vi "main003.vi"() -> ()   [LabVIEW 2015]
uses:
  <vilib>/DAQmx/write.llb/DAQmx Write (Analog DBL 1Chan 1Samp).vi
  <vilib>/DAQmx/miscellaneous.llb/DAQmx Fill In Error Info.vi
  <vilib>/DAQmx/create/channels.llb/DAQmx Create Channel (AO-Voltage-Basic).vi
  subvi/Newport ESP301/Newport ESP301.lvlib
panel:
  out "speed":dbl(graph)
  in  "pump_waypoints":string[][](table)
  in  "Boolean":bool
  out "a":waveform(dbl)(graph)={"t0"=timestamp(3620209335.8073797 s since 1904-01-01), "dt"=1.0, "Y"=[nan]}
  out "Waveform Chart":dbl(graph)=5.25341140860948
  in  "physical channels":tag="Dev3/ao1"
  out "DAC error":errorcluster
  out "ESP error":errorcluster={"status"=TRUE, "code"=-1073807343, "source"="VISA Open in Newport ESP301.lvlib:Initialize.vi->main002.vi"}
  out "run?":bool
  in  "set_vel":bool
  in  "velocity [fs/s]":dbl=667.128190396304
  in  "vel_mm":dbl caption="velocity [mm/s]"
  out "meas. velocity":dbl=nan
  in  "stop":bool
  out "output voltage":dbl=nan
  in  "start":bool
  in  "go2p1":bool
  out "position [fs]":dbl=nan
  out "position [mm]":dbl=nan
  in  "p2 [mm]":dbl=2.0
  in  "p1 [mm]":dbl
  in  "interpolate output":bool
  in  "t2 [fs]":dbl=6671.281903963041
  in  "t1 [fs]":dbl=-6671.281903963041
  in  "t0 [mm]":dbl=1.0
  in  "Axis (1)":i32=2 min=1 max=3
  in  "Serial Link (RS232)":enum16{"RS232", "USB"}(ring)
  in  "VISA resource name":refnum<visa-resource-name>="COM9"
  in  "main_close":bool
  # "Always use CLOSE button to correctly disconnect the device. STOP program afterwards."
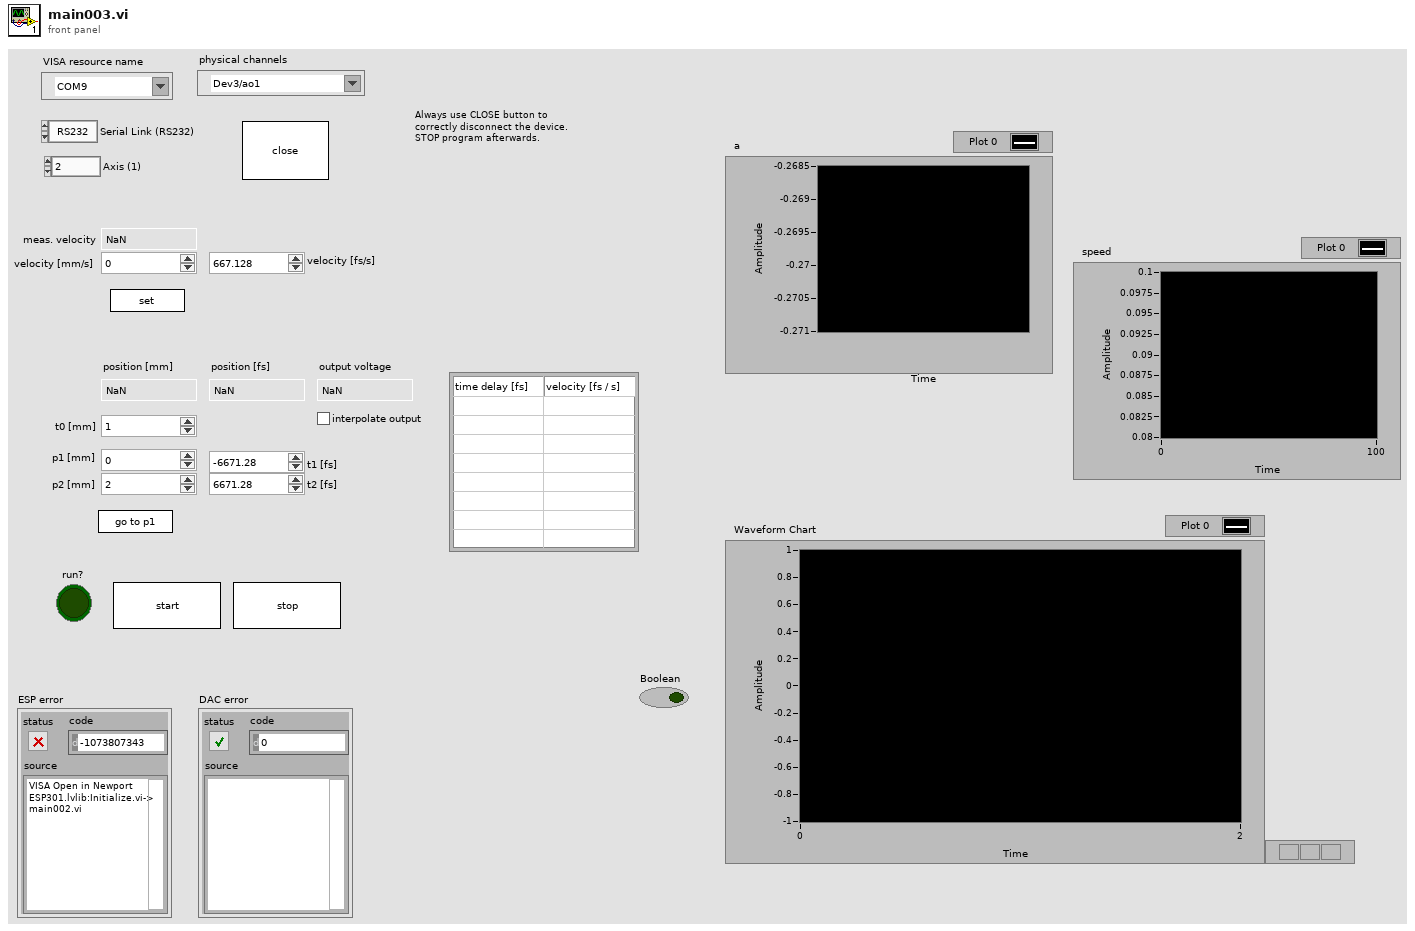
[diagram p1: front panel]
types:
  T1 = cluster{"dev1_data":refnum<queue>, "dev2_data":refnum<queue>}
  T2 = cluster{"dev1_cmd":refnum<queue>, "dev2_cmd":refnum<queue>}
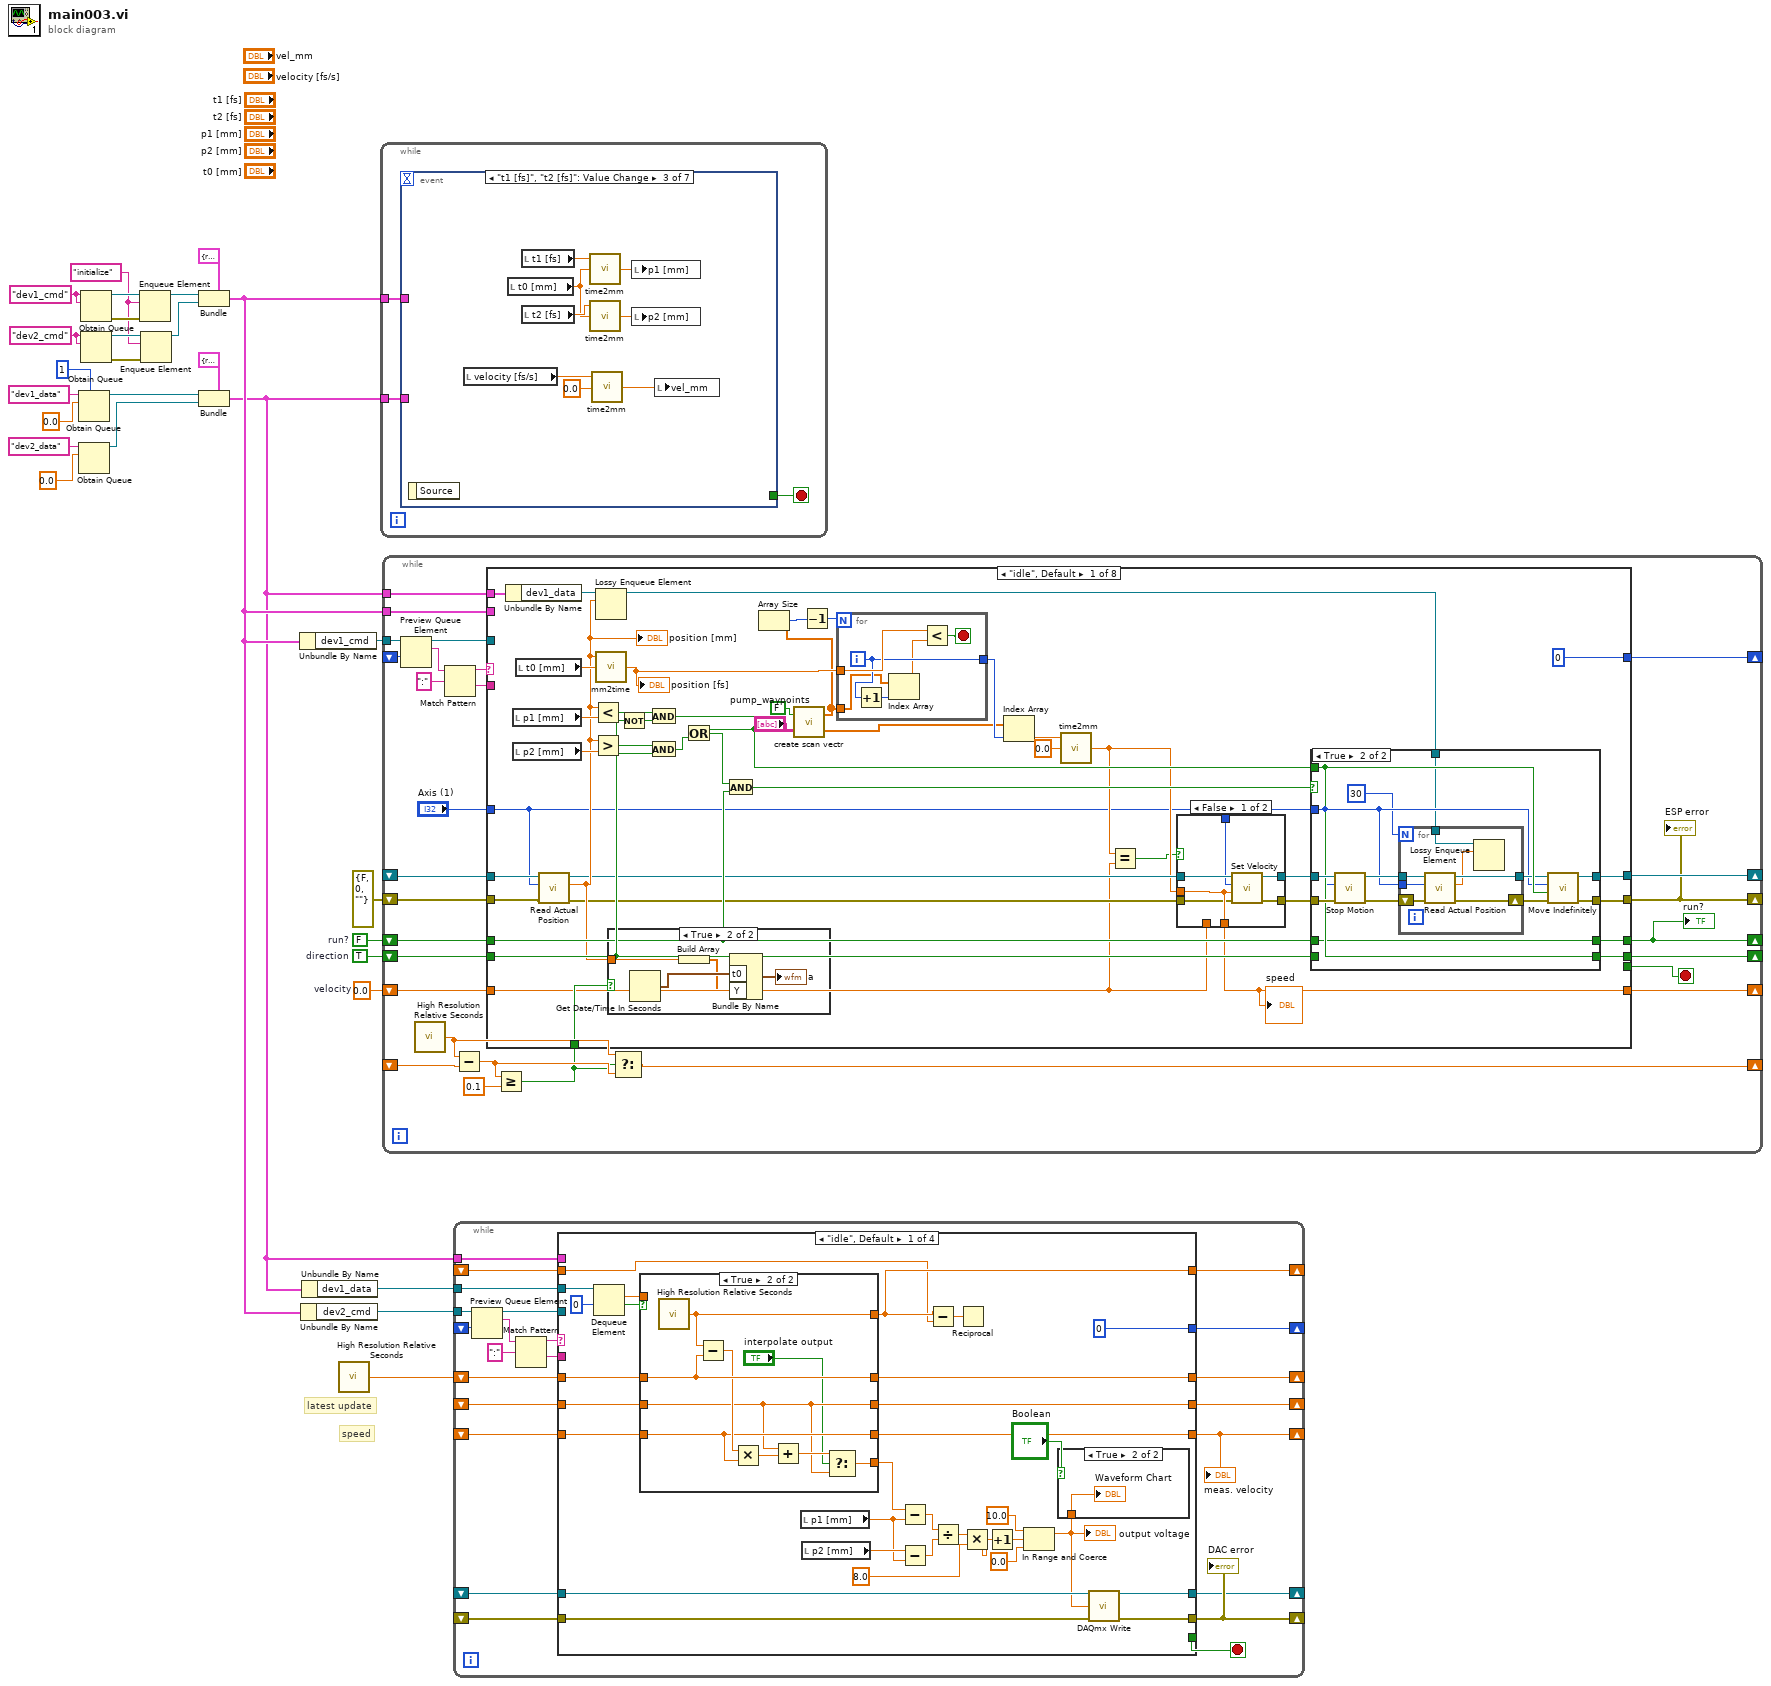
[diagram p0: block diagram]
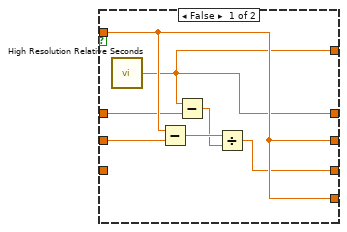
[diagram p3: hidden frame]
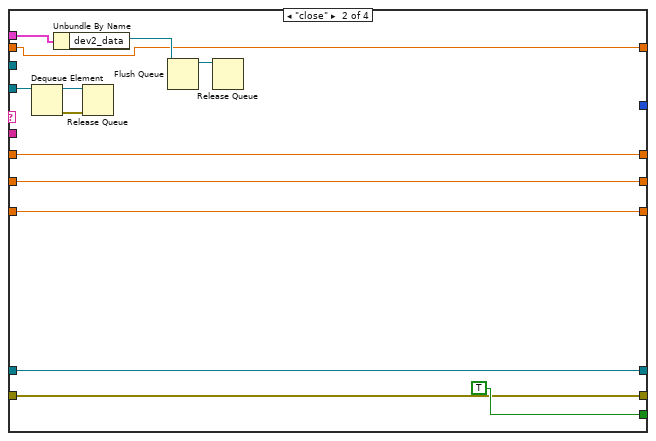
[diagram p4: hidden frame]
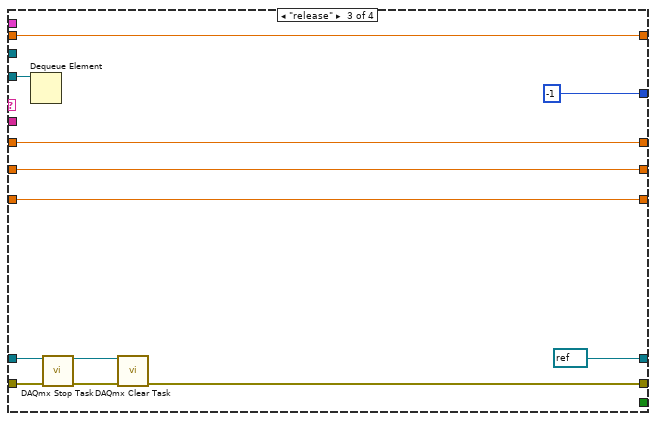
[diagram p5: hidden frame]
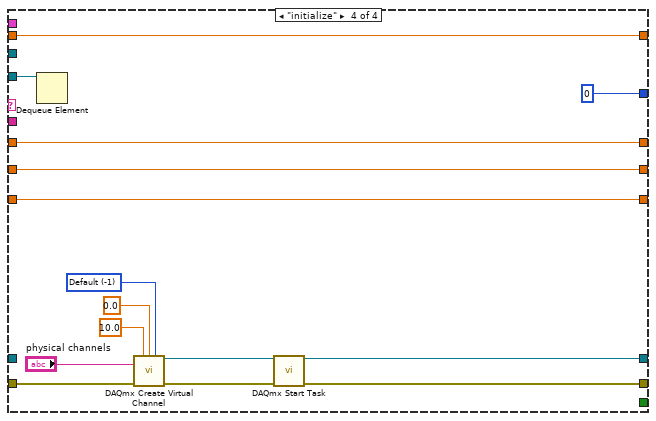
[diagram p6: hidden frame]
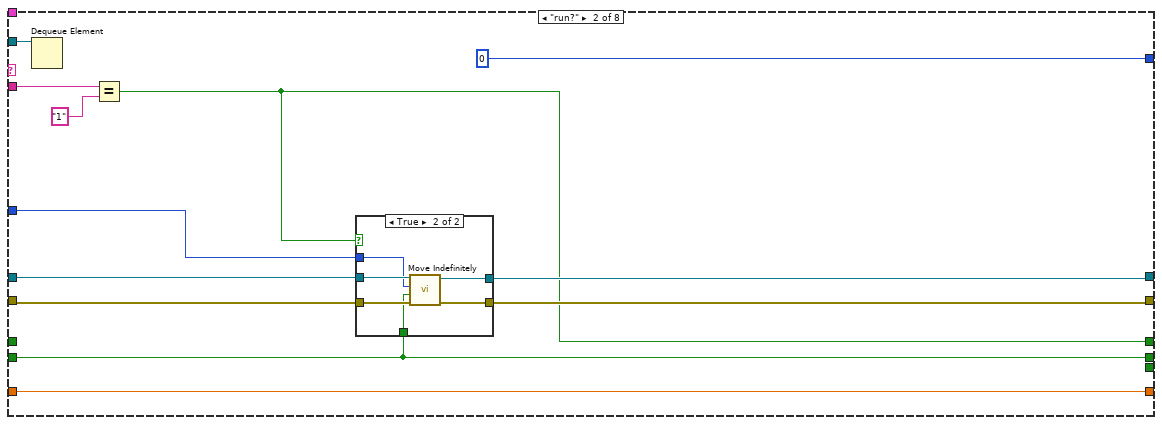
[diagram p10: hidden frame]
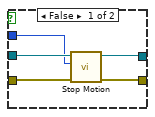
[diagram p11: hidden frame]
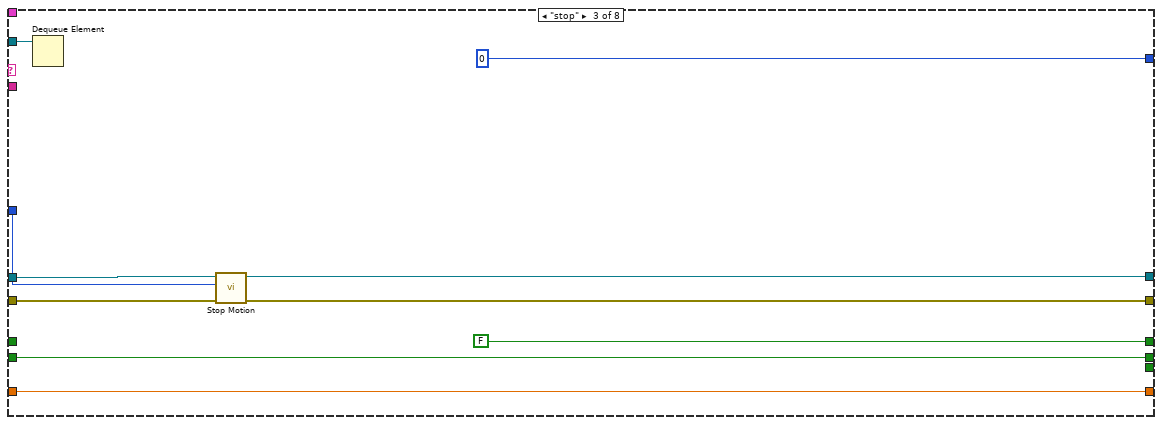
[diagram p12: hidden frame]
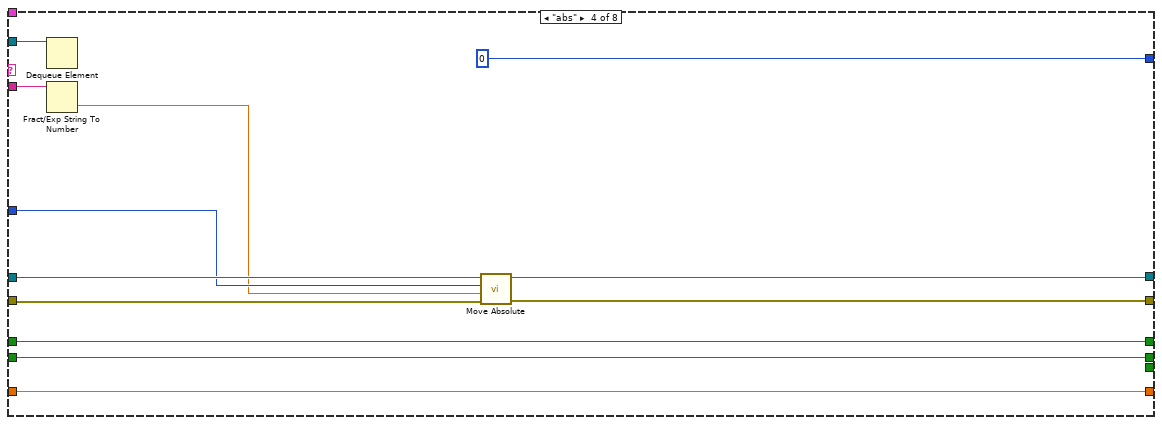
[diagram p13: hidden frame]
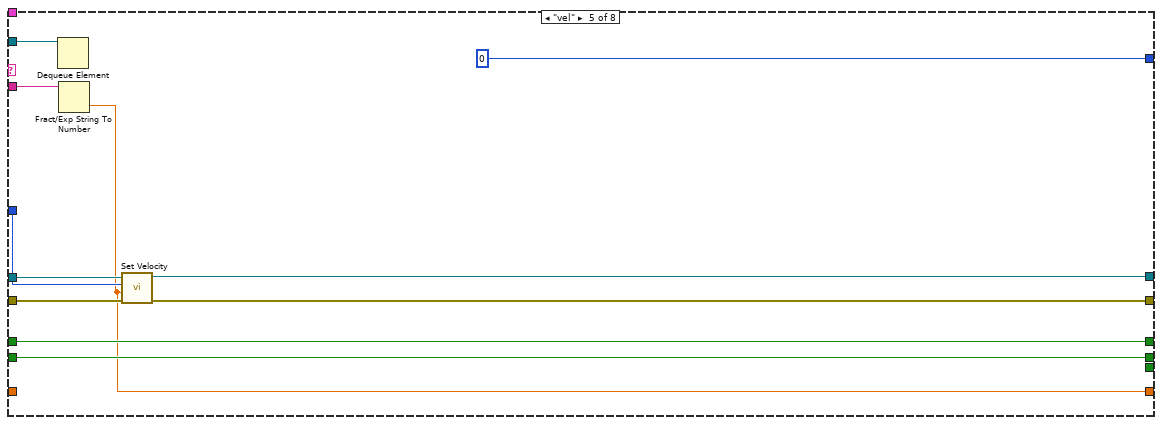
[diagram p14: hidden frame]
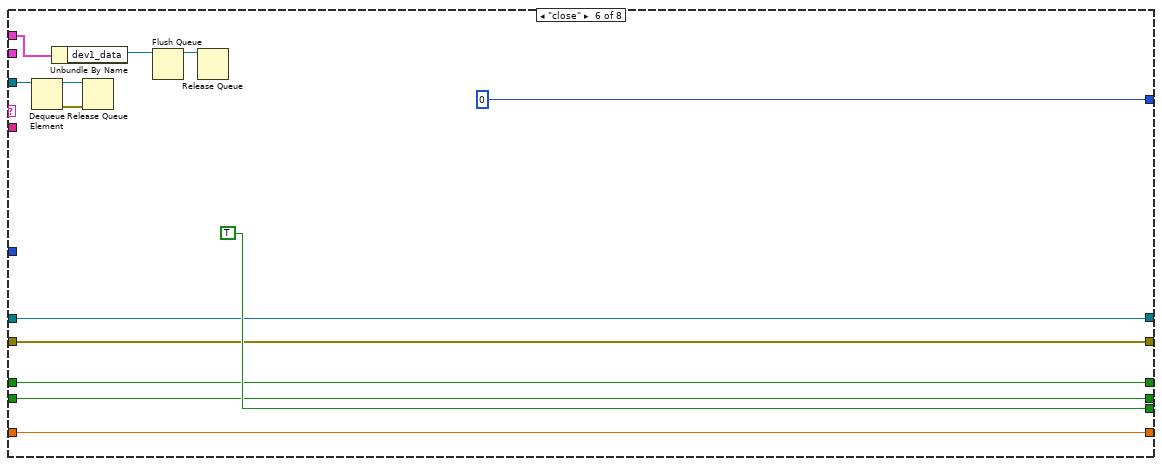
[diagram p15: hidden frame]
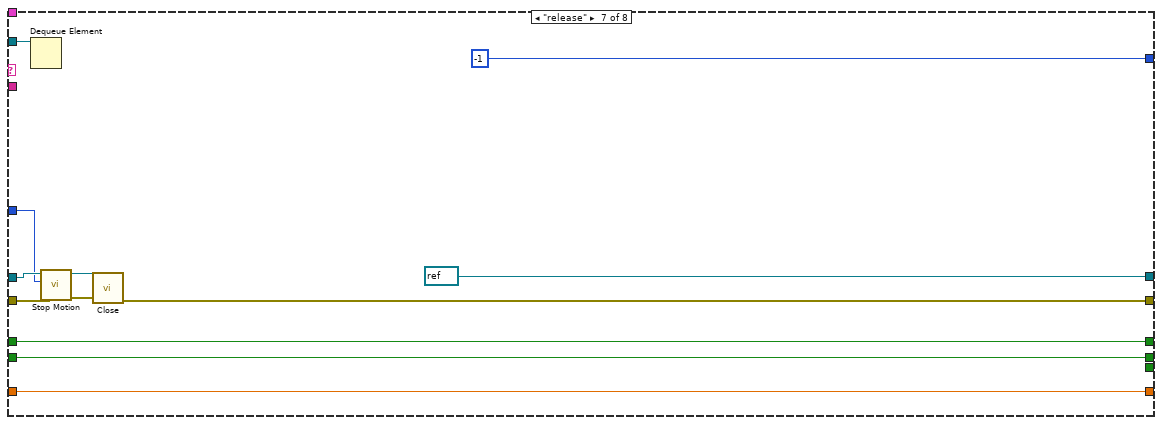
[diagram p16: hidden frame]
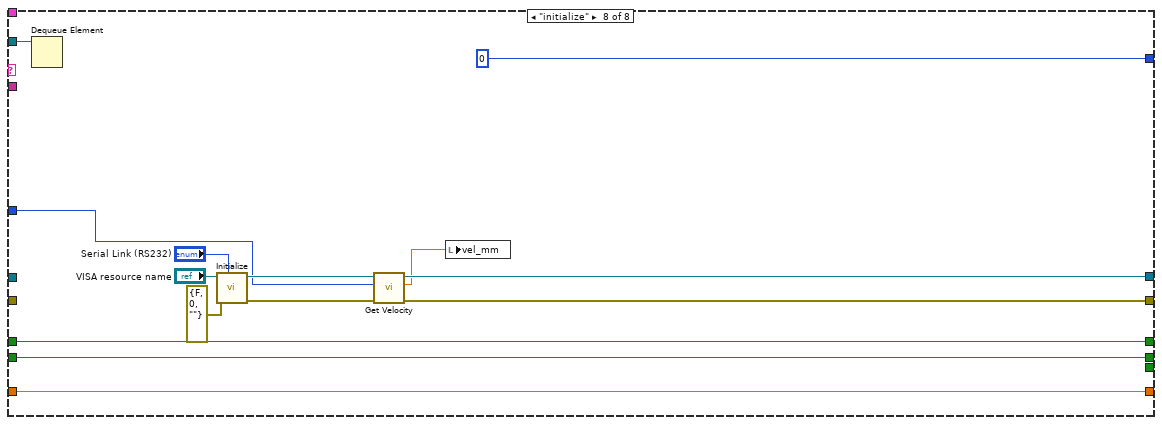
[diagram p17: hidden frame]
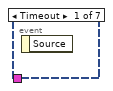
[diagram p18: hidden frame]
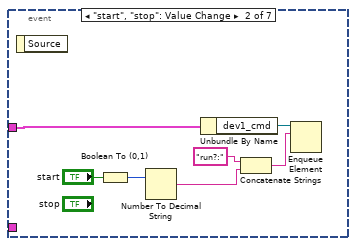
[diagram p19: hidden frame]
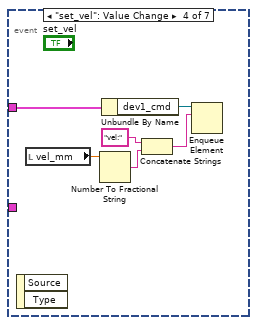
[diagram p20: hidden frame]
diagram:
  w1 = 0.0  # velocity
  w2 = TRUE  # direction
  w5 = FALSE  # run?
  w16 = "dev2_cmd" ("name (unnamed)")
  w22 = "initialize" ("element")
  w17 = "dev1_cmd" ("name (unnamed)")
  # "speed"
  # "latest update"
  n1 = Obtain Queue(max queue size (-1, unlimited)=1, name (unnamed)="dev1_data", element data type=0.0) -> (queue out=w13:refnum<queue>)  [unwired: 2 in, 2 out]
  n2 = Obtain Queue(name (unnamed)="dev2_data", element data type=0.0) -> (queue out=w12:refnum<queue>)  [unwired: 3 in, 2 out]
  n3 = Obtain Queue(name (unnamed)=w17, element data type=w17) -> (queue out=w28:refnum<queue>, error out=w27:errorcluster)  [unwired: 3 in, 1 out]
  n4 = Obtain Queue(name (unnamed)=w16, element data type=w16) -> (queue out=w23:refnum<queue>, error out=w24:errorcluster)  [unwired: 3 in, 1 out]
  n5 = Enqueue Element(queue=w28, element=w22, error in (no error)=w27) -> (queue out=w25:refnum<queue>)  [unwired: 1 in, 2 out]
  n6 = Enqueue Element(queue=w23, element=w22, error in (no error)=w24) -> (queue out=w21:refnum<queue>)  [unwired: 1 in, 2 out]
  n7 = Bundle(cluster=T2 {"dev1_cmd"=refnum, "dev2_cmd"=refnum}, "dev1_cmd"=w25, "dev2_cmd"=w21) -> (w9:T2)
  n8 = Bundle(cluster=T1 {"dev1_data"=refnum, "dev2_data"=refnum}, "dev1_data"=w13, "dev2_data"=w12) -> (w3:T1)
  n9 = Unbundle By Name(w9) -> ("dev1_cmd"=w18:refnum<queue>)
  n10 = Unbundle By Name(w9) -> ("dev2_cmd"=w8:refnum<queue>)
  n11 = Unbundle By Name(w3) -> ("dev1_data"=w7:refnum<queue>)
  n12 = call <vilib>:"High Resolution Relative Seconds.vi"() -> ("relative seconds"=w6:dbl)
  n13 = while {
    tunnel: w9 -> [w31]
    tunnel: w3 -> [w30]
    stop <- w29 stop-if-true
    n14 = event shown="[2] \"t1 [fs]\", \"t2 [fs]\": Value Change" {
      selector: _ -> [_ _ _ _ _ _ _]
      dyn-events: _ -> [_ _ _ _ _ _ _]
      timeout: _ -> [_ _ _ _ _ _ _]
      tunnel: w31 -> [_ w35 _ w48 _ w66 w69]
      tunnel: w30 -> [_ _ _ _ _ _ _]
      tunnel: [_ _ _ _ _ _ TRUE] -> w29
      event Timeout {
        n15 = event-data() -> ()  [unwired: 1 in, 1 out]
      }
      event "start", "stop": Value Change {
        n16 = event-data() -> ()  [unwired: 1 in, 1 out]
        n17 = Boolean To (0,1)(Boolean="start") -> (0, 1=w33:i16)
        n18 = Number To Decimal String(number=w33) -> (decimal integer string=w32:string)  [unwired: 1 in]
        n19 = Unbundle By Name(w35) -> ("dev1_cmd"=w38:refnum<queue>)
        n20 = Concatenate Strings("run?:" ("string"), w32) -> (w37:string)
        n21 = Enqueue Element(queue=w38, element=w37) -> ()  [unwired: 2 in, 3 out]
      }
      event "t1 [fs]", "t2 [fs]": Value Change {
        n22 = event-data() -> ()  [unwired: 1 in, 1 out]
        n23 = local read "velocity [fs/s]"() -> (w41:dbl)
        n24 = local read "t0 [mm]"() -> (w44:dbl)
        n25 = local read "t1 [fs]"() -> (w45:dbl)
        n26 = local read "t2 [fs]"() -> (w46:dbl)
        n27 = call "time2mm.vi"("Offset (mm)"=w44, "time"=w45) -> ("position (mm)"=w42:dbl)  [unwired: 1 in]
        n28 = call "time2mm.vi"("Offset (mm)"=w44, "time"=w46) -> ("position (mm)"=w43:dbl)  [unwired: 1 in]
        n29 = call "time2mm.vi"("Offset (mm)"=0.0, "time"=w41) -> ("position (mm)"=w39:dbl)  [unwired: 1 in]
        n30 = local write "p1 [mm]"(w42) -> ()
        n31 = local write "p2 [mm]"(w43) -> ()
        n32 = local write "vel_mm"(w39) -> ()
      }
      event "set_vel": Value Change {
        n33 = event-data() -> ()  [unwired: 1 in, 2 out]
        n34 = local read "vel_mm"() -> (w47:dbl)
        n35 = Number To Fractional String(number=w47) -> (F-format string=w51:string)  [unwired: 3 in]
        n36 = Unbundle By Name(w48) -> ("dev1_cmd"=w52:refnum<queue>)
        n37 = Concatenate Strings("vel:" ("string"), w51) -> (w50:string)
        n38 = Enqueue Element(queue=w52, element=w50) -> ()  [unwired: 2 in, 3 out]
      }
      event "p1 [mm]", "p2 [mm]", "t0 [mm]", "vel_mm": Value Change {
        n39 = event-data() -> ()  [unwired: 1 in, 2 out]
        n40 = local read "vel_mm"() -> (w55:dbl)
        n41 = local read "p1 [mm]"() -> (w59:dbl)
        n42 = local read "p2 [mm]"() -> (w60:dbl)
        n43 = local read "t0 [mm]"() -> (w58:dbl)
        n44 = call "mm2time.vi"("Offset (mm)"=w58, "distance (mm)"=w59) -> ("time in fs"=w56:dbl)  [unwired: 1 in]
        n45 = call "mm2time.vi"("Offset (mm)"=w58, "distance (mm)"=w60) -> ("time in fs"=w57:dbl)  [unwired: 1 in]
        n46 = call "mm2time.vi"("Offset (mm)"=0.0, "distance (mm)"=w55) -> ("time in fs"=w54:dbl)  [unwired: 1 in]
        n47 = local write "t1 [fs]"(w56) -> ()
        n48 = local write "t2 [fs]"(w57) -> ()
        n49 = local write "velocity [fs/s]"(w54) -> ()
      }
      event "go2p1": Value Change {
        n50 = event-data() -> ()  [unwired: 1 in, 2 out]
        n51 = local read "p1 [mm]"() -> (w61:dbl)
        n52 = Number To Fractional String(number=w61) -> (F-format string=w64:string)  [unwired: 3 in]
        n53 = Unbundle By Name(w66) -> ("dev1_cmd"=w65:refnum<queue>)
        n54 = Concatenate Strings("abs:" ("string"), w64) -> (w62:string)
        n55 = Enqueue Element(queue=w65, element=w62) -> ()  [unwired: 2 in, 3 out]
      }
      event "main_close": Value Change {
        n56 = event-data() -> ()  [unwired: 1 in, 1 out]
        n57 = Cluster To Array(cluster=w69) -> (array=w68:refnum<queue>[])
        n58 = for {
          tunnel: w68 -> [w74] mode=indexing
          n59 = Flush Queue(queue=w74) -> (queue out=w70:refnum<queue>)  [unwired: 1 in, 2 out]
          n60 = Enqueue Element(queue=w70, element="release") -> (queue out=w72:refnum<queue>)  [unwired: 2 in, 2 out]
          n61 = Enqueue Element(queue=w72, element="close") -> ()  [unwired: 2 in, 3 out]
        }
      }
    }
  }
  n62 = while {
    tunnel: w9 -> [w97]
    tunnel: w18 -> [w102]
    tunnel: w3 -> [w94]
    shift-right: [w92] -> _
    shift-left: _ -> [w93]
    shift-right: [w91] -> _
    shift-left: _ -> [w88]
    shift-right: [w90] -> _
    shift-left: errorcluster {"status"=FALSE, "code"=0, "source"=""} ("error out") -> [w89]
    shift-right: [w85] -> _
    shift-left: w5 -> [w86]
    shift-right: [w83] -> _
    shift-left: w2 -> [w84]
    shift-right: [w77] -> _
    shift-left: _ -> [w82]
    shift-right: [w75] -> _
    shift-left: w1 -> [w76]
    stop <- w95 stop-if-true
    n63 = Preview Queue Element(queue=w102, timeout in ms (-1)=w93) -> (queue out=w96:refnum<queue>, element=w101:string)  [unwired: 1 in, 2 out]
    n64 = call <vilib>:"High Resolution Relative Seconds.vi"() -> ("relative seconds"=w79:dbl)
    n65 = Match Pattern(string=w101, regular expression=":") -> (before substring=w99:string, after substring=w98:string)  [unwired: 1 in, 2 out]
    n66 = Subtract(x=w79, y=w82) -> (x-y=w80:dbl)
    n67 = Greater Or Equal?(x=w80, y=0.1) -> (x >= y?=w78:bool)
    n68 = case shown="\"idle\", Default" w99 {
      tunnel: w98 -> [_ w200 _ w232 w239 _ _ _]
      tunnel: w97 -> [_ _ _ _ _ _ _ _]
      tunnel: w96 -> [_ w198 w214 w233 w238 w257 w268 w279]
      tunnel: [_ _ _ _ _ TRUE _ _] -> w95
      tunnel: w94 -> [w144 _ _ _ _ w249 _ _]
      tunnel: [0 0 0 0 0 0 -1 0] -> w92
      tunnel: [w119 w195 w219 w229 w244 w253 refnum<visa-resource-name> refnum ("VISA resource name out") w275] -> w91
      tunnel: [w114 w194 w218 w228 w243 w252 w267 w274] -> w90
      tunnel: w89 -> [w140 w192 w220 w230 w242 w252 w263 _]
      tunnel: w88 -> [w141 w193 w221 w231 w241 w253 w260 _]
      tunnel: "Axis (1)" -> [w108 w196 w217 w227 w240 _ w259 w276]
      tunnel: w86 -> [w129 _ _ w224 w236 w250 w265 w280]
      tunnel: [w128 w191 FALSE ("run?") w224 w236 w250 w265 w280] -> w85
      tunnel: w84 -> [w130 w190 w213 w223 w235 w246 w264 w271]
      tunnel: [w131 w190 w213 w223 w235 w246 w264 w271] -> w83
      tunnel: w78 -> [w127 _ _ _ _ _ _ _]
      tunnel: w76 -> [w113 w189 w212 w222 _ w245 w258 w270]
      tunnel: [w106 w189 w212 w222 w234 w245 w258 w270] -> w75
      frame "idle", Default {
        n69 = Unbundle By Name(w144) -> ("dev1_data"=w143:refnum<queue>)
        n70 = local read "p1 [mm]"() -> (w139:dbl)
        n71 = local read "p2 [mm]"() -> (w138:dbl)
        n72 = local read "t0 [mm]"() -> (w142:dbl)
        n73 = call "Read Actual Position.vi"("error in (no error)"=w140, "Axis (1)"=w108, "VISA resource name"=w141) -> ("error out"=w115:errorcluster, "Position (units)"=w126:dbl, "VISA resource name out"=w118:refnum<visa-resource-name>)  [unwired: 2 in]
        "position [mm]" <- w126
        n74 = Less?(x=w126, y=w139) -> (x < y?=w136:bool)
        n75 = Greater?(x=w126, y=w138) -> (0:w135:bool)
        n76 = Lossy Enqueue Element(queue=w143, element=w126) -> (queue out=w125:refnum<queue>)  [unwired: 1 in, 3 out]
        n77 = call "mm2time.vi"("Offset (mm)"=w142, "distance (mm)"=w126) -> ("time in fs"=w120:dbl)  [unwired: 1 in]
        "position [fs]" <- w120
        n78 = case shown="True" w127 {
          tunnel: w126 -> [_ w164]
          frame False {
          }
          frame True {
            n79 = Get Date/Time In Seconds() -> (seconds since 1Jan1904=w163:timestamp)
            n80 = Build Array(w164) -> (w162:dbl[])
            n81 = Bundle By Name("t0"=w163, "Y"=w162) -> (→"a":waveform(dbl))  [unwired: 1 in]
          }
        }
        n82 = Not(x=w130) -> (.not. x?=w137:bool)
        n83 = And(x=w136, y=w137) -> (x .and. y?=w132:bool)
        n84 = And(x=w135, y=w130) -> (x .and. y?=w134:bool)
        n85 = Or(x=w132, y=w134) -> (x .or. y?=w133:bool)
        n86 = And(x=w133, y=w129) -> (x .and. y?=w112:bool)
        n87 = call "create scan vectr.vi"("Table Control"="pump_waypoints", "waypoint mode?"=FALSE) -> ("Array 2"=w123:dbl[], "Array"=w105:dbl[])
        n88 = Array Size(array=w105) -> (size(s)=w103:i32)
        n89 = Decrement(x=w103) -> (x-1=w104:i32)
        n90 = for {
          N: w104 -> [_]
          tunnel: w105 -> [w155]
          tunnel: w120 -> [w160]
          tunnel: [w157] -> w124
          i -> [w157]
          stop <- w159 stop-if-true
          n91 = Increment(x=w157) -> (x+1=w158:i32)
          n92 = Index Array(array=w155, index=w158) -> (element=w156:dbl)
          n93 = Less?(x=w160, y=w156) -> (x < y?=w159:bool)
        }
        n94 = Index Array(array=w123, index=w124) -> (element=w111:dbl)
        n95 = call "time2mm.vi"("Offset (mm)"=0.0, "time"=w111) -> ("position (mm)"=w109:dbl)  [unwired: 1 in]
        n96 = Equal?(x=w109, y=w113) -> (x = y?=w107:bool)
        n97 = case shown="False" w107 {
          tunnel: w118 -> [w148 w154]
          tunnel: [w151 w154] -> w117
          tunnel: [w150 w153] -> w116
          tunnel: w115 -> [w146 w153]
          tunnel: w113 -> [_ w152]
          tunnel: [w149 w152] -> w106
          tunnel: w109 -> [w149 _]
          tunnel: w108 -> [w147 _]
          frame False {
            n98 = call "Set Velocity.vi"("error in (no error)"=w146, "Velocity (units/s)"=w149, "Axis (1)"=w147, "VISA resource name"=w148) -> ("error out"=w150:errorcluster, "VISA resource name out"=w151:refnum<visa-resource-name>)  [unwired: 2 in]
          }
          frame True {
          }
        }
        "speed" <- w106
        n99 = case shown="True" w112 {
          tunnel: w117 -> [w168 w179]
          tunnel: w116 -> [w167 w178]
          tunnel: [w168 w181] -> w119
          tunnel: [w167 w180] -> w114
          tunnel: w108 -> [_ w171]
          tunnel: w132 -> [_ w177]
          tunnel: [w166 w177] -> w131
          tunnel: w130 -> [w166 _]
          tunnel: w129 -> [w165 w176]
          tunnel: [w165 w176] -> w128
          tunnel: w125 -> [_ w170]
          frame False {
          }
          frame True {
            n100 = call "Stop Motion.vi"("error in (no error)"=w178, "Axis (1)"=w171, "VISA resource name"=w179) -> ("error out"=w173:errorcluster, "VISA resource name out"=w175:refnum<visa-resource-name>)  [unwired: 3 in]
            n101 = for {
              N: 30 -> [_]
              tunnel: w175 -> [w188]
              tunnel: [w187] -> w174
              shift-right: [w185] -> w172
              shift-left: w173 -> [w186]
              tunnel: w171 -> [w184]
              tunnel: w170 -> [w183]
              n102 = call "Read Actual Position.vi"("error in (no error)"=w186, "Axis (1)"=w184, "VISA resource name"=w188) -> ("error out"=w185:errorcluster, "Position (units)"=w182:dbl, "VISA resource name out"=w187:refnum<visa-resource-name>)  [unwired: 2 in]
              n103 = Lossy Enqueue Element(queue=w183, element=w182) -> ()  [unwired: 1 in, 4 out]
            }
            n104 = call "Move Indefinitely.vi"("error in (no error)"=w172, "Move Direction (+)"=w177, "Axis (1)"=w171, "VISA resource name"=w174) -> ("error out"=w180:errorcluster, "VISA resource name out"=w181:refnum<visa-resource-name>)  [unwired: 2 in]
          }
        }
      }
      frame "run?" {
        n105 = Dequeue Element(queue=w198) -> ()  [unwired: 2 in, 4 out]
        n106 = Equal?(x=w200, y="1") -> (x = y?=w191:bool)
        n107 = case shown="True" w191 {
          tunnel: w193 -> [w205 w211]
          tunnel: w192 -> [w202 w210]
          tunnel: w196 -> [w201 w209]
          tunnel: [w204 w208] -> w195
          tunnel: [w203 w207] -> w194
          tunnel: w190 -> [_ w206]
          frame False {
            n108 = call "Stop Motion.vi"("error in (no error)"=w202, "Axis (1)"=w201, "VISA resource name"=w205) -> ("error out"=w203:errorcluster, "VISA resource name out"=w204:refnum<visa-resource-name>)  [unwired: 3 in]
          }
          frame True {
            n109 = call "Move Indefinitely.vi"("error in (no error)"=w210, "Move Direction (+)"=w206, "Axis (1)"=w209, "VISA resource name"=w211) -> ("error out"=w207:errorcluster, "VISA resource name out"=w208:refnum<visa-resource-name>)  [unwired: 2 in]
          }
        }
      }
      frame "stop" {
        n110 = Dequeue Element(queue=w214) -> ()  [unwired: 2 in, 4 out]
        n111 = call "Stop Motion.vi"("error in (no error)"=w220, "Axis (1)"=w217, "VISA resource name"=w221) -> ("error out"=w218:errorcluster, "VISA resource name out"=w219:refnum<visa-resource-name>)  [unwired: 3 in]
      }
      frame "abs" {
        n112 = Dequeue Element(queue=w233) -> ()  [unwired: 2 in, 4 out]
        n113 = Fract/Exp String To Number(string=w232) -> (number=w226:dbl)  [unwired: 3 in, 1 out]
        n114 = call "Move Absolute.vi"("error in (no error)"=w230, "Position (0 units)"=w226, "Axis (1)"=w227, "VISA resource name"=w231) -> ("error out"=w228:errorcluster, "VISA resource name out"=w229:refnum<visa-resource-name>)  [unwired: 2 in]
      }
      frame "vel" {
        n115 = Dequeue Element(queue=w238) -> ()  [unwired: 2 in, 4 out]
        n116 = Fract/Exp String To Number(string=w239) -> (number=w234:dbl)  [unwired: 3 in, 1 out]
        n117 = call "Set Velocity.vi"("error in (no error)"=w242, "Velocity (units/s)"=w234, "Axis (1)"=w240, "VISA resource name"=w241) -> ("error out"=w243:errorcluster, "VISA resource name out"=w244:refnum<visa-resource-name>)  [unwired: 2 in]
      }
      frame "close" {
        n118 = Dequeue Element(queue=w257) -> (queue out=w256:refnum<queue>, error out=w255:errorcluster)  [unwired: 2 in, 2 out]
        n119 = Unbundle By Name(w249) -> ("dev1_data"=w247:refnum<queue>)
        n120 = Release Queue(queue=w256, error in (no error)=w255) -> ()  [unwired: 1 in, 3 out]
        n121 = Flush Queue(queue=w247) -> (queue out=w248:refnum<queue>)  [unwired: 1 in, 2 out]
        n122 = Release Queue(queue=w248) -> ()  [unwired: 2 in, 3 out]
      }
      frame "release" {
        n123 = Dequeue Element(queue=w268) -> ()  [unwired: 2 in, 4 out]
        n124 = call "Stop Motion.vi"("error in (no error)"=w263, "Axis (1)"=w259, "VISA resource name"=w260) -> ("error out"=w262:errorcluster, "VISA resource name out"=w261:refnum<visa-resource-name>)  [unwired: 3 in]
        n125 = call "Close.vi"("error in (no error)"=w262, "VISA resource name"=w261) -> ("error out"=w267:errorcluster)  [unwired: 9 in]
      }
      frame "initialize" {
        n126 = Dequeue Element(queue=w279) -> ()  [unwired: 2 in, 4 out]
        n127 = call "Initialize.vi"("VISA resource name"="VISA resource name", "error in (no error)"=errorcluster {"status"=FALSE, "code"=0, "source"=""}, "Serial Link (RS232)"="Serial Link (RS232)") -> ("VISA resource name out"=w278:refnum<visa-resource-name>, "error out"=w277:errorcluster)  [unwired: 6 in]
        n128 = call "Get Velocity.vi"("error in (no error)"=w277, "Axis (1)"=w276, "VISA resource name"=w278) -> ("error out"=w274:errorcluster, "Velocity (units/s)"=w273:dbl, "VISA resource name out"=w275:refnum<visa-resource-name>)  [unwired: 2 in]
        n129 = local write "vel_mm"(w273) -> ()
      }
    }
    "run?" <- w85
    "ESP error" <- w90
    n130 = Select(t=w79, s=w78, f=w80) -> (s? t:f=w77:dbl)
  }
  n131 = while {
    shift-right: [w299] -> _
    shift-left: _ -> [w300]
    shift-right: [w298] -> _
    shift-left: _ -> [w297]
    tunnel: w8 -> [w296]
    shift-right: [w295] -> _
    shift-left: _ -> [w294]
    tunnel: w7 -> [w293]
    shift-right: [w292] -> _
    shift-left: _ -> [w289]
    shift-right: [w291] -> _
    shift-left: w6 -> [w290]
    shift-right: [w284] -> _
    shift-left: _ -> [w288]
    tunnel: w3 -> [w287]
    shift-right: [w286] -> _
    shift-left: _ -> [w285]
    stop <- w301 stop-if-true
    n132 = Preview Queue Element(queue=w296, timeout in ms (-1)=w300) -> (queue out=w302:refnum<queue>, element=w306:string)  [unwired: 1 in, 2 out]
    n133 = Match Pattern(string=w306, regular expression=":") -> (before substring=w304:string, after substring=w303:string)  [unwired: 1 in, 2 out]
    n134 = case shown="\"idle\", Default" w304 {
      tunnel: w303 -> [_ _ _ _]
      tunnel: w302 -> [_ w367 w378 w386]
      tunnel: [_ TRUE _ _] -> w301
      tunnel: [0 _ -1 0] -> w299
      tunnel: [w333 w363 w377 w387] -> w298
      tunnel: w297 -> [w331 w363 w374 w394]
      tunnel: [w334 w362 refnum<k21> refnum ("task out") w388] -> w295
      tunnel: w294 -> [w332 w362 w375 _]
      tunnel: w293 -> [w335 _ _ _]
      tunnel: [w329 w360 w370 w383] -> w292
      tunnel: [w328 w361 w371 w384] -> w291
      tunnel: w290 -> [w326 w361 w371 w384]
      tunnel: w289 -> [w327 w360 w370 w383]
      tunnel: [w325 w359 w369 w382] -> w284
      tunnel: w288 -> [w324 w359 w369 w382]
      tunnel: w287 -> [_ w356 _ _]
      tunnel: [w313 w355 w368 w380] -> w286
      tunnel: w285 -> [w312 w355 w368 w380]
      frame "idle", Default {
        n135 = Dequeue Element(queue=w335, timeout in ms (-1)=0) -> (element=w330:dbl, timed out?=w314:bool)  [unwired: 1 in, 2 out]
        n136 = case shown="True" w314 {
          tunnel: w330 -> [w345 _]
          tunnel: [w345 w347] -> w323
          tunnel: [w345 w349] -> w329
          tunnel: [w339 w354] -> w328
          tunnel: w327 -> [w344 w349]
          tunnel: w326 -> [w343 w354]
          tunnel: [w340 w351] -> w325
          tunnel: w324 -> [_ w351]
          tunnel: [w339 w346] -> w313
          frame False {
            n137 = call <vilib>:"High Resolution Relative Seconds.vi"() -> ("relative seconds"=w339:dbl)
            n138 = Subtract(x=w345, y=w344) -> (x-y=w342:dbl)
            n139 = Subtract(x=w339, y=w343) -> (x-y=w341:dbl)
            n140 = Divide(x=w342, y=w341) -> (x/y=w340:dbl)
          }
          frame True {
            n141 = call <vilib>:"High Resolution Relative Seconds.vi"() -> ("relative seconds"=w346:dbl)
            n142 = Subtract(x=w346, y=w354) -> (x-y=w353:dbl)
            n143 = Multiply(x=w353, y=w351) -> (x*y=w352:dbl)
            n144 = Add(x=w349, y=w352) -> (x+y=w350:dbl)
            n145 = Select(t=w350, s="interpolate output", f=w349) -> (s? t:f=w347:dbl)
          }
        }
        n146 = local read "p1 [mm]"() -> (w321:dbl)
        n147 = local read "p2 [mm]"() -> (w322:dbl)
        n148 = Subtract(x=w323, y=w321) -> (x-y=w320:dbl)
        n149 = Subtract(x=w322, y=w321) -> (x-y=w319:dbl)
        n150 = Subtract(x=w313, y=w312) -> (x-y=w311:dbl)
        n151 = Divide(x=w320, y=w319) -> (x/y=w318:dbl)
        n152 = Reciprocal(x=w311) -> ()  [unwired: 1 out]
        n153 = Multiply(x=w318, y=8.0) -> (x*y=w309:dbl)
        n154 = Increment(x=w309) -> (x+1=w308:dbl)
        n155 = In Range and Coerce(upper limit=10.0, x=w308, lower limit=0.0) -> (coerced(x)=w310:dbl)  [unwired: 1 out]
        "output voltage" <- w310
        n156 = case shown="True" "Boolean" {
          tunnel: w310 -> [_ w338]
          frame False {
          }
          frame True {
            "Waveform Chart" <- w338
          }
        }
        n157 = call-poly <vilib>:"DAQmx Write.vi"("task/channels in"=w332, "data"=w310, "error in"=w331) -> ("task out"=w334:refnum<k21>, "error out"=w333:errorcluster)  [unwired: 10 in, 1 out]
      }
      frame "close" {
        n158 = Dequeue Element(queue=w367) -> (queue out=w366:refnum<queue>, error out=w365:errorcluster)  [unwired: 2 in, 2 out]
        n159 = Unbundle By Name(w356) -> ("dev2_data"=w357:refnum<queue>)
        n160 = Release Queue(queue=w366, error in (no error)=w365) -> ()  [unwired: 1 in, 3 out]
        n161 = Flush Queue(queue=w357) -> (queue out=w358:refnum<queue>)  [unwired: 1 in, 2 out]
        n162 = Release Queue(queue=w358) -> ()  [unwired: 2 in, 3 out]
      }
      frame "release" {
        n163 = Dequeue Element(queue=w378) -> ()  [unwired: 2 in, 4 out]
        n164 = call <vilib>:"DAQmx Stop Task.vi"("task/channels in"=w375, "error in"=w374) -> ("task out"=w373:refnum<k21>, "error out"=w372:errorcluster)  [unwired: 12 in]
        n165 = call <vilib>:"DAQmx Clear Task.vi"("task in"=w373, "error in"=w372) -> ("error out"=w377:errorcluster)  [unwired: 13 in]
      }
      frame "initialize" {
        w391 = -1 items=["Default"=-1, "RSE"=10083, "Differential"=10106, "Pseudodifferential"=12529] ("output terminal configuration")
        n166 = Dequeue Element(queue=w386) -> ()  [unwired: 2 in, 4 out]
        n167 = call-poly <vilib>:"DAQmx Create Virtual Channel.vi"("maximum value"=10.0, "minimum value"=0.0, "output terminal configuration"=w391, "physical channels"="physical channels", "error in"=w394) -> ("task out"=w390:refnum<k21>, "error out"=w389:errorcluster)  [unwired: 9 in]
        n168 = call <vilib>:"DAQmx Start Task.vi"("task/channels in"=w390, "error in"=w389) -> ("task out"=w388:refnum<k21>, "error out"=w387:errorcluster)  [unwired: 12 in]
      }
    }
    "meas. velocity" <- w284
    "DAC error" <- w298
  }
